vi "Area in Loop.vi"(8 "error in (no error)":errorcluster, 11 "Map in":refnum<class "Maze.lvclass">) -> (0 "error out":errorcluster, 2 "Area":u64, 3 "Map out":refnum<class "Maze.lvclass">)   [LabVIEW 2021, in "Maze.lvclass"]
uses:
  Maze.lvclass
  Maze.lvclass/Maze.ctl
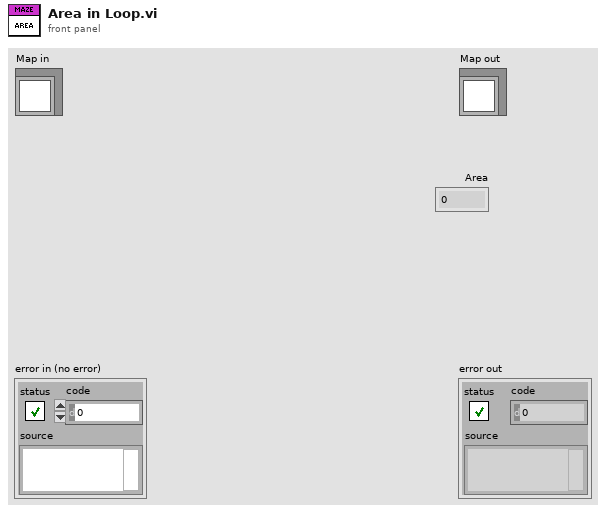
[diagram p1: front panel]
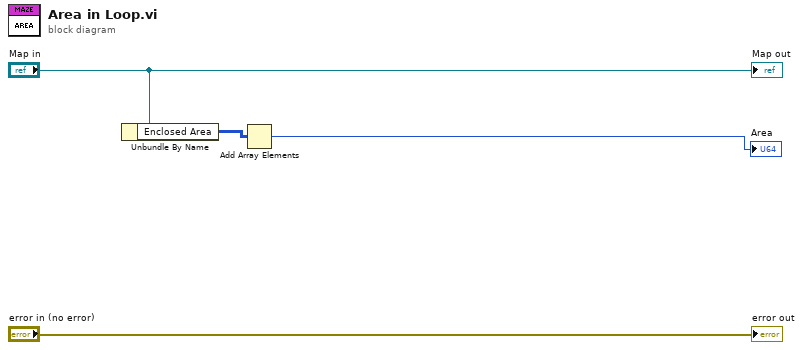
[diagram p0: block diagram]
diagram:
  n1 = Unbundle By Name("Map in") -> ("Enclosed Area"=w2:i32[][])
  n2 = Add Array Elements(numeric array=w2) -> (sum=→"Area":i32)
  "error out" <- "error in (no error)"
  "Map out" <- "Map in"
